vi "Send Close View FP.vi"(7 "Priority":T1=enum."Normal" caption="Message Priority (Normal)", 8 "error in (no error)":errorcluster, 9 "View Hierarchy Level":i32, 10 "View":string, 11 "Message Enqueuer in":refnum<class "Message Enqueuer.lvclass">) -> (0 "error out":errorcluster, 3 "Message Enqueuer out":refnum<class "Message Enqueuer.lvclass">)   [LabVIEW 2023, in "GUI Views.lvlib" / "Close View FP Msg.lvclass"]
doc: "Sends the <b>GUI Views.lvlib:Close View FP Msg.lvclass</b> message.\n\nThis message will call <b>Close View FP.vi</b> on the <b>GUI Views.lvlib:GUI Container Actor.lvclass</b> actor.\n\n<b>Close View FP.vi Description</b>\nCloses the Front Panel of a specified Actor Core VI of the the specified View class hierarchy. The Front Panel is specified by: \n\n<b> View </b> String theat contains the name of the View\n\n<b> View Hierarchy Level</b> the level on the subclassing hierarchy of the GUI View actor, it is used to choose the Actor Core Front Panel among all the exisiting sublcasses of the GUI VIew Actor present in the View specified above"
uses:
  Close View FP Msg.lvclass
  Close View FP Msg.lvclass/Close View FP Msg.ctl
  <vilib>/ActorFramework/Message Enqueuer/Message Enqueuer.lvclass
  C:/Program Files/National Instruments/LabVIEW 2023/vi.lib/ActorFramework/Message/Message.lvclass
  C:/Projects/Shared Libraries/Event Actors/GUI Views/GUI Container Actor Messages/Close View FP Msg/Close View FP Msg.lvclass
  <vilib>/ActorFramework/Message Enqueuer/Message Priority.ctl
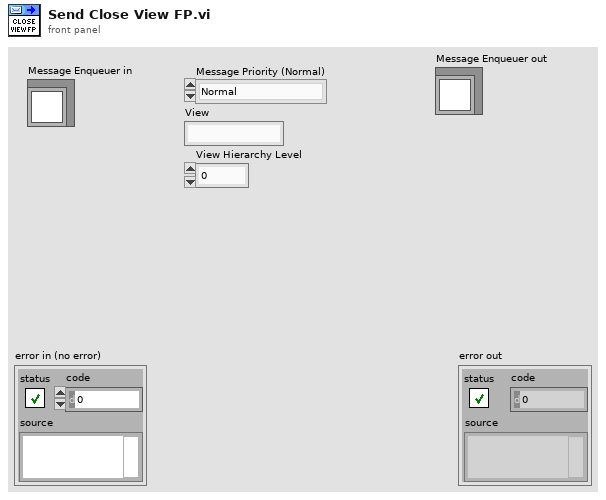
[diagram p1: front panel]
types:
  T1 = typedef "Actor Framework.lvlib/Message Enqueuer.lvclass/Message Priority.ctl" = enum16{"Low", "Normal", "High"}
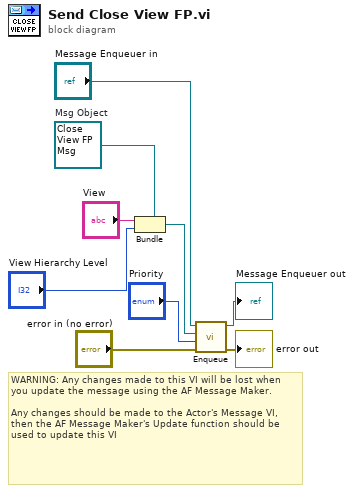
[diagram p0: block diagram]
diagram:
  w7 = refnum<class "Close View FP Msg.lvclass"> refnum  # Msg Object
  # "WARNING: Any changes made to this VI will be lost when you update the message using the AF Message Maker.\n\nAny changes should be made to the Actor's Message VI, then the AF Message Maker's Update function should be used to update this VI"
  n1 = Bundle(cluster=w7, "View", "View Hierarchy Level") -> (w2:refnum<class "Close View FP Msg.lvclass">)
  n2 = call <vilib>:"Enqueue.vi"("error in (no error)"="error in (no error)", "Message Priority (Normal)"="Priority", "Message"=w2, "Message Enqueuer in"="Message Enqueuer in") -> ("error out"=→"error out":errorcluster, "Message Enqueuer out"=→"Message Enqueuer out":refnum<class "Message Enqueuer.lvclass">)  [unwired: 6 in]
